vi "DHE_CalcMinExpTime.vi"(10 "calculated value in (s)":dbl, 11 "Database RefNum out":T1) -> (1 "min_exp_time(ms)":dbl, 2 "min_exp_time(s)":dbl)   [LabVIEW 2016]
uses:
  DBSHAND/private/vis/DatabaseHand_RefNum.ctl
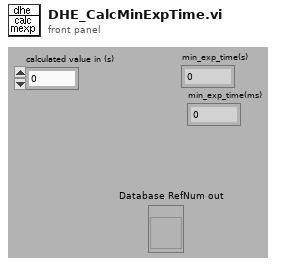
[diagram p1: front panel]
types:
  T1 = typedef "DatabaseHand_RefNum.ctl" = refnum<vi>
  T2 = typedef "CMN_TimingInfo.ctl" = cluster{"PixelTime":sgl, "SkipPixel":sgl, "SkipRow":sgl, "ShiftRow":sgl, "ShiftedPix":u16, "known_overhead":sgl, "DET_READ_TIME":sgl}
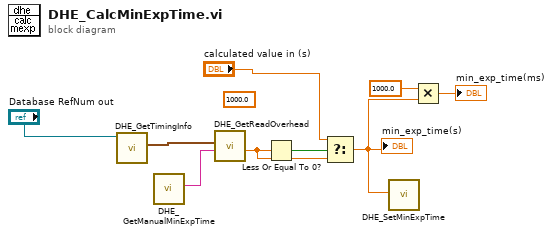
[diagram p0: block diagram]
diagram:
  (unwired) 1000.0 ("y")
  n1 = call "DHE_GetTimingInfo.vi"("Database RefNum out"="Database RefNum out") -> ("Timing"=w8:T2)  [unwired: 10 out]
  n2 = call "DHE_GetManualMinExpTime.vi"() -> ("ManualMinExpTime"=w7:string)  [unwired: 11 out]
  n3 = call "DHE_GetReadOverhead.vi"("overhead string"=w7, "Timing"=w8) -> ("overhead"=w5:dbl)  [unwired: 9 out]
  n4 = Less Or Equal To 0?(x=w5) -> (x <= 0?=w6:bool)
  n5 = Select(t="calculated value in (s)", s=w6, f=w5) -> (s? t:f=w4:dbl)
  "min_exp_time(s)" <- w4
  n6 = call "DHE_SetMinExpTime.vi"("MinExpTime"=w4) -> ()  [unwired: 11 out]
  n7 = Multiply(x=1000.0, y=w4) -> (x*y=→"min_exp_time(ms)":dbl)
